vi "Calculate Constants.vi"(1 "Z":dbl, 2 "Y":dbl, 3 "X":dbl) -> (0 "constants cluster":cluster{"a":dbl, "b":dbl, "c":dbl, "d":dbl})   [LabVIEW 2016]
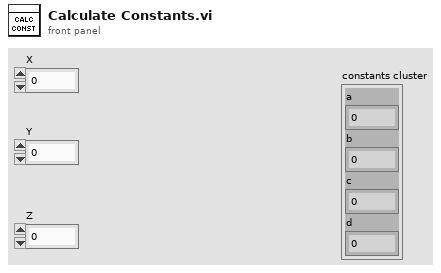
[diagram p1: front panel]
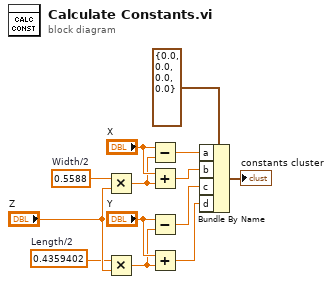
[diagram p0: block diagram]
diagram:
  w6 = 0.4359402  # Length/2
  w8 = 0.5588  # Width/2
  n1 = Multiply(x=w8, y="Z") -> (x*y=w1:dbl)
  n2 = Multiply(x=w6, y="Z") -> (x*y=w3:dbl)
  n3 = Subtract(x="X", y=w1) -> (x-y=w10:dbl)
  n4 = Add(x="X", y=w1) -> (x+y=w7:dbl)
  n5 = Subtract(x="Y", y=w3) -> (x-y=w5:dbl)
  n6 = Add(x="Y", y=w3) -> (x+y=w2:dbl)
  n7 = Bundle By Name(cluster=cluster{"a":dbl, "b":dbl, "c":dbl, "d":dbl} {"a"=0.0, "b"=0.0, "c"=0.0, "d"=0.0}, "a"=w10, "b"=w7, "c"=w5, "d"=w2) -> (→"constants cluster":cluster{"a":dbl, "b":dbl, "c":dbl, "d":dbl})
